vi "PTP.vi"(2 "Run uninterrupted?":bool, 3 "Device Category IN:":string(combo)="Mini" caption="Device Category:", 5 "Sensor Serial No. IN:":string caption="Sensor Serial No.:", 6 "DB Serial No. IN:":string caption="DB Serial No.:") -> (0 "Done!":bool)   [LabVIEW 2019]
doc: "Performs IV measurements according to ATLAS ITk Quality Control Specifications."
uses:
  general_VIs/globals/QC_MeasurementSetup.vi
  general_VIs/globals/QC_RunInformation.vi
  InstrControl/InstrumentSetup.vi
  InstrControl/Switching/Switching.lvclass
  InstrControl/SupplyControl/SupplyControl.lvclass
  InstrControl/ArduinoControl/ArduinoControl.lvclass
  InstrControl/InstrControl.lvclass
  <vilib>/Analysis/NI_AALBase.lvlib
panel:
  out "Measurement Configuration Tab":enum32{"PTP Setup", "PTP Scan"}(tab)
  in  "Test step [V] IN":dbl=10.0 caption="Test Step [V]" format="%.1f"
  in  "Set current limits?":bool
  in  "Current Limit Bias [µA]":dbl=1000.0 min=0.0001 format="%.3f"
  in  "Measurement Configurations":bool
  in  "Bias Voltage [V] IN":dbl=-700.0 caption="Bias Voltage [V]"
  in  "Bias step [V] IN":dbl=10.0 caption="Bias Step [V]" format="%.1f"
  in  "step interval [s] IN":i32=10 caption="Step Interval [s]"
  in  "Continue":bool
  in  "Quit":bool
  in  "Test Final Voltage [V] IN":dbl=-700.0 caption="Test Final Voltage [V]"
  in  "Current Limit SMU [µA]":dbl=1000.0 min=0.0001 format="%.3f"
  out "RH":dbl[](array[numeric]) caption="RH [%]" format="%#.2f"
  out "Temp.":dbl[](array[numeric]) caption="Temp. [°C]" format="%#.2f"
  out "R_eff":dbl[](array[numeric]) caption="Current [nA]"
  out "Volts":dbl[](array[numeric]) caption="Volts [V]"
  out "step interval [s]":i32=10
  out "step [V]":dbl=10.0 format="%.1f"
  out "Final volts [V]":dbl=-700.0 format="%.1f"
  out "Initial volts [V]":dbl format="%.1f"
  out "Igraph":cluster{dbl[], dbl[]}(graph)
  in  "Scales":T1(ring)
  in  "Iscale":enum16{"Ohms", "kiloOhms", "MegaOhms"}(ring)
  out "positive ramp?":bool
  out "DUT Description/Hardware Tab":enum32{"PTP Setup", "PTP Scan"}(tab)
  in  "Structure  Name IN:":string caption="Stucture Name:"
  in  "Test SMU":string(combo)="Keithley 2657A"
  in  "Switching":string(combo)="LXIPXI Switching"
  in  "Hardware Configurations":bool
  in  "User:":string(combo)="Xavi"
  in  "Bias Supply":string(combo)="Keithley 2410"
  in  "Temperature":enum16{"Read Arduino", "Enter manually"}(ring)
  in  "Manufacturer:":string(combo)="Hamamatsu"
  out "Structure Name:":string
  in  "abort":bool
  out "Device Category:":string
  out "DB Serial No.:":string
  out "Current Volts:":dbl format="%.2f"
  in  "quit (no save)":bool
  in  "Quit & Save":bool
  out "Bias On/Off:":bool
  out "STATUS 1":string
  out "Initiated:":string
  out "Sensor No.:":string
  out "No of steps":u32
  out "Current reading No.":u32
  out "Last reading at:":string
  # "Vertical Scale:"
  # "Strip Sensor Testing: PTP"
  # "Measurement Configuration"
  # "PTP Scan parameters:"
  # "Last 5 readings:"
  # "n-4"
  # "n-3"
  # "n-2"
  # "n-1"
  # "n"
  # "DUT Description"
  # "Hardware"
  # "DUT & Test Description:"
  # "Current status:"
  # "Rdg No:"
  # "out of"
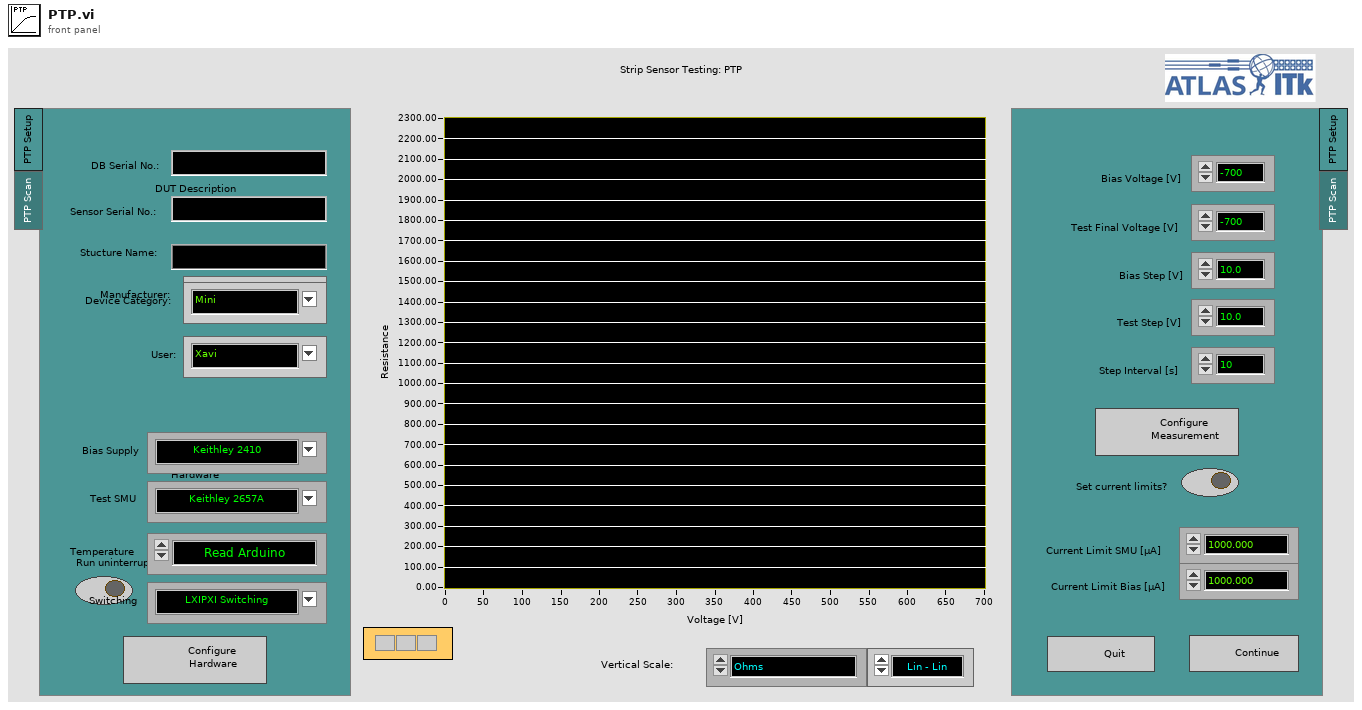
[diagram p1: front panel]
types:
  T1 = enum16{"Lin - Lin", "Log - Lin", "Lin - Log", "Log - log"}
  T2 = enum16{"Supply", "LCR", "Multimeter", "Switching"}
  T3 = enum16{"Reset", "Read Array", "Read Element", "Write Element", "Write Array", "Add Element", "Add Array"}
  T4 = enum16{"Reset", "Ground", "Striptest Bias", "Striptest SMU", "Striptest LCR", "IV", "CV", "Interstrip Cap", "Interstrip Res"}
  T5 = enum16{"Reset", "Ground", "Striptest Bias", "Striptest SMU", "Striptest LCR", "IV", "CV", "Interstrip Cap", "Interstrip Res", "PTP", "Implant Resistance", "Metal Resistance", "Coupling Capacitance"}
  T6 = cluster{"Supply":refnum<class "SupplyControl.lvclass">, "Final Test Voltage [V]":dbl, "Bias Voltage [V]":dbl, "Bias Step Size [V]":dbl, "Step Interval [s]":i32, "Bias Number of Steps":u32, "Ramp down steps [V]":dbl, "Ramp down Interval [s]":i32, "Set Current Limit?":bool, "Current Limit Bias [µA]":dbl, "Temperature Readout":enum16{"Read Arduino", "Enter manually"}, "Arduino":refnum<class "ArduinoControl.lvclass">, "Supply Name":string, "V_breakdown Limit [V]":dbl, "Switching":refnum<class "Switching.lvclass">, "Matrix used?":bool, "Matrix X Channels":cluster{"Bias Supply / SMU LO":i32, "Bias Supply / SMU HI":i32, "CV Box LO":i32, "CV Box HI":i32, "CV Box LO IN":i32, "CV Box HI IN":i32, "Volt meter LO":i32, "Volt meter HI":i32, "Mux1 C1":i32, "Mux1 C2":i32, "Mux2 C1":i32, "Mux2 C2":i32}, "SMU Name":string, "Test Step Size [V] ":dbl, "Test Number of Steps ":u32, "SMU":refnum<class "SupplyControl.lvclass">, "Current Limit SMU [µA] ":dbl, "Structure Name":string}
  T7 = cluster{"Sensor Serial No.:":string, "Wafer Serial No.:":string, "Batch:":string, "Manufacturer:":string, "Device Category:":string, "Database Serial No.:":string, "Date Initiated:":string, "Time Initiated:":string, "Test":string, "Instruments used:":string, "Probeplan used:":string, "End of Run comment:":string, "User:":string}
  T8 = cluster{"Institute":string, "Manufacturers":string[], "Devices":string[], "Serialnumbers Lookup DB":string, "Data directory":string, "Backup & screenshot directory":string, "List of known users":string[], "Measurement switch not used":bool, "Measurement Switch":string, "DUT Switch":string}
  T9 = cluster{"Current Limit":sgl, "KE2410":refnum<class "KE2410.lvclass">}
  T10 = cluster{"Current Limit":sgl, "KE2657A":refnum<class "KE2657A.lvclass">}
  T11 = cluster{"VISA address":refnum<visa-resource-name>, "T sensor":enum16{"SHT", "DS"}, "Arduino":refnum<class "ArduinoControl.lvclass">}
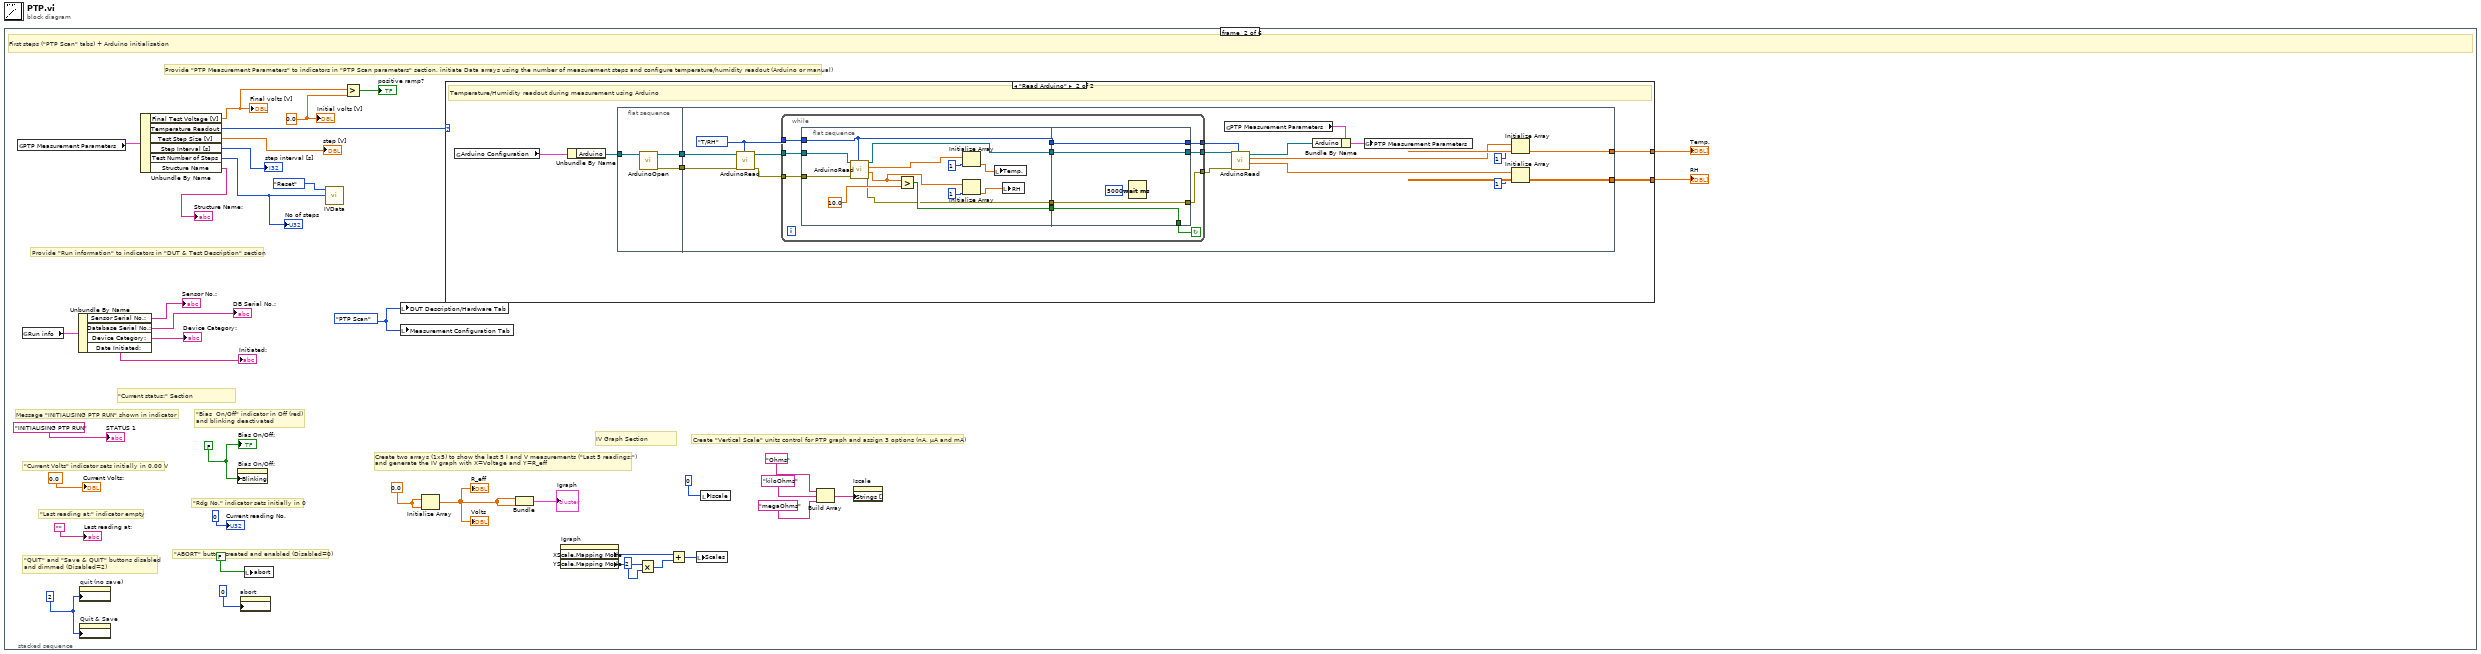
[diagram p0: block diagram]
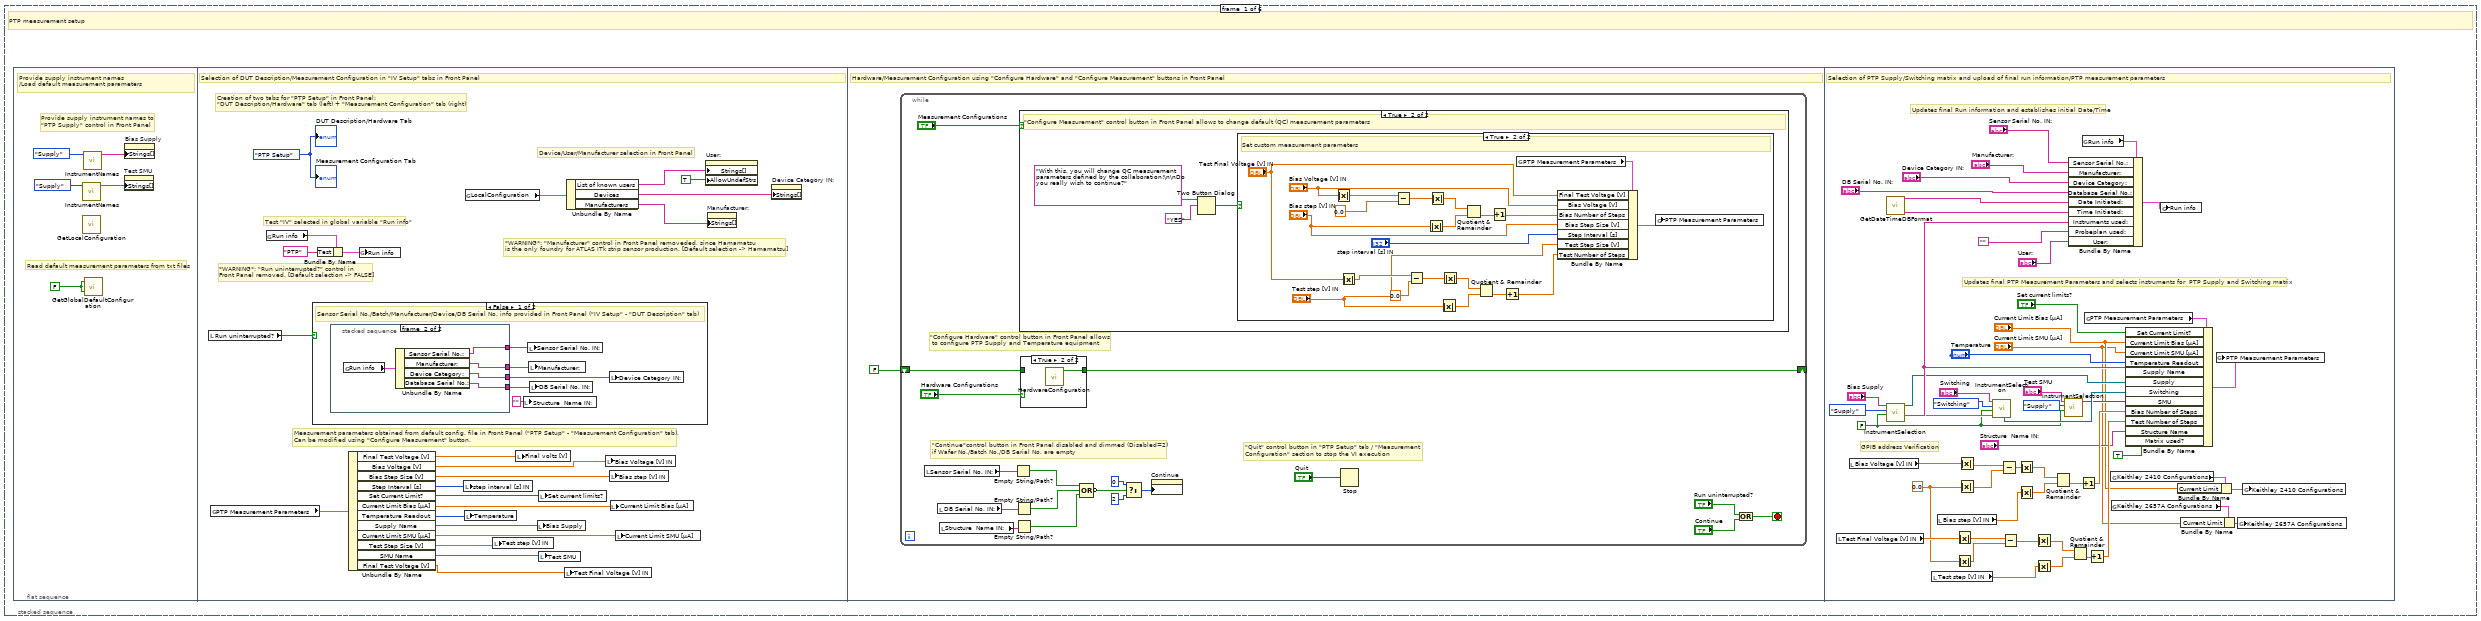
[diagram p2: hidden frame]
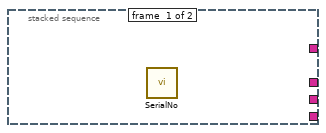
[diagram p3: hidden frame]
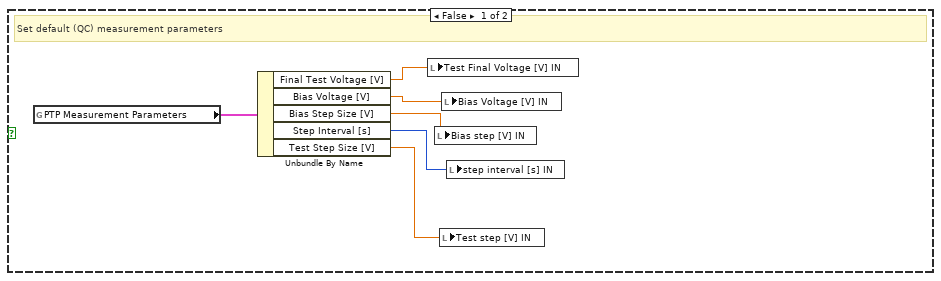
[diagram p6: hidden frame]
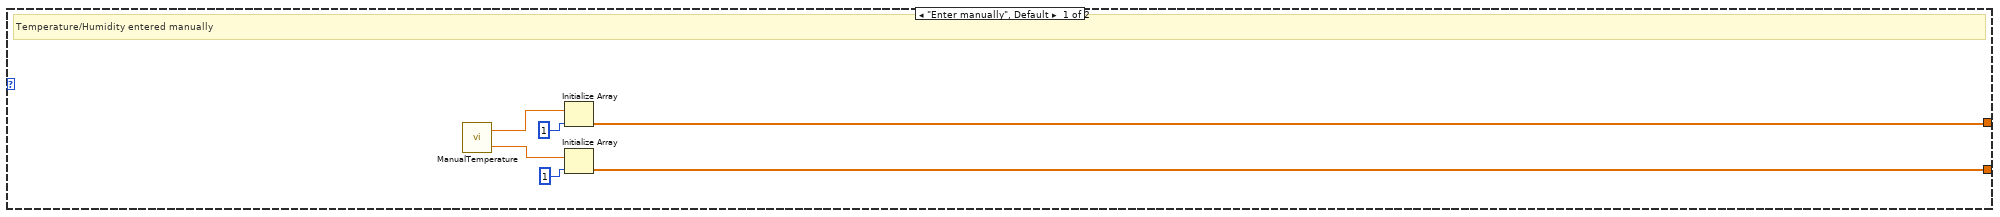
[diagram p8: hidden frame]
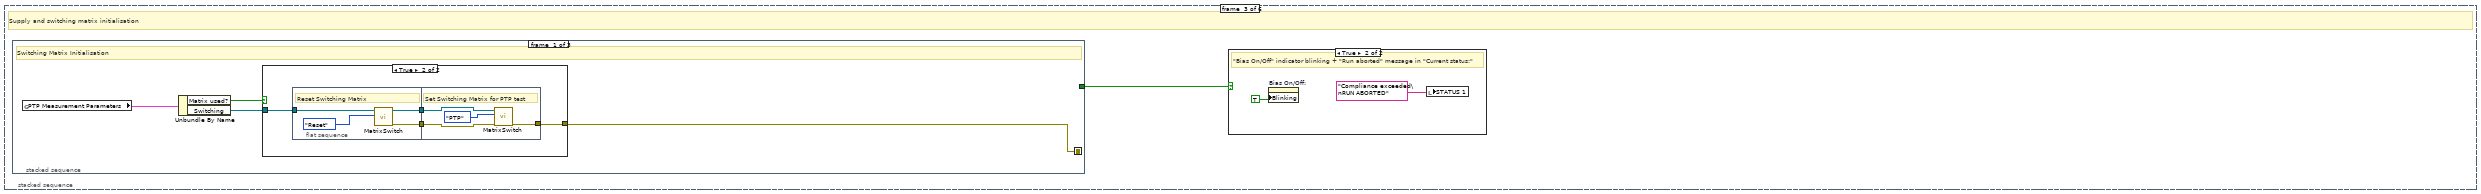
[diagram p9: hidden frame]
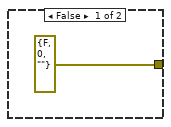
[diagram p10: hidden frame]
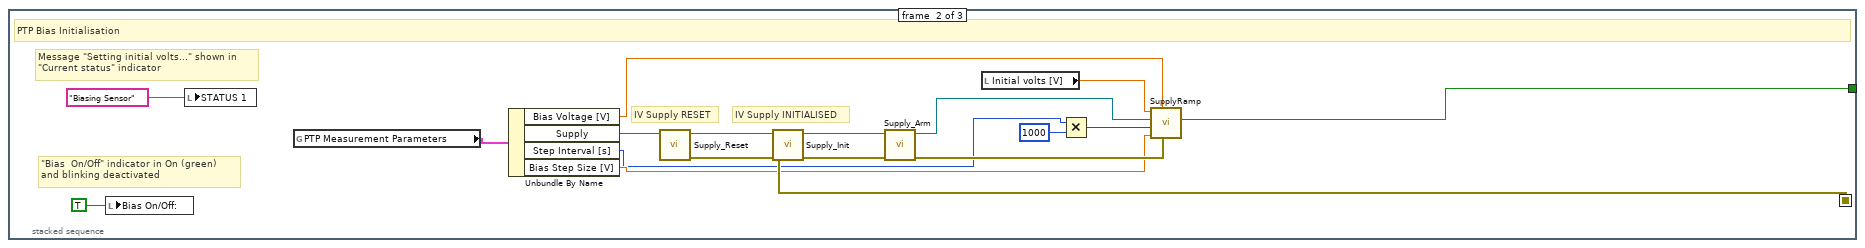
[diagram p11: hidden frame]
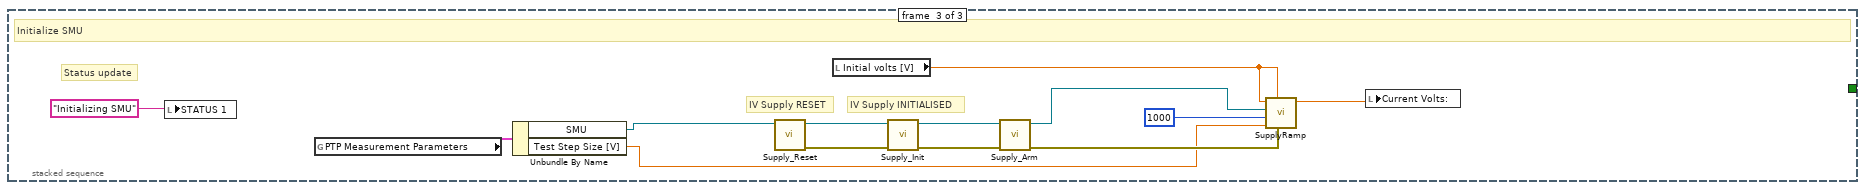
[diagram p12: hidden frame]
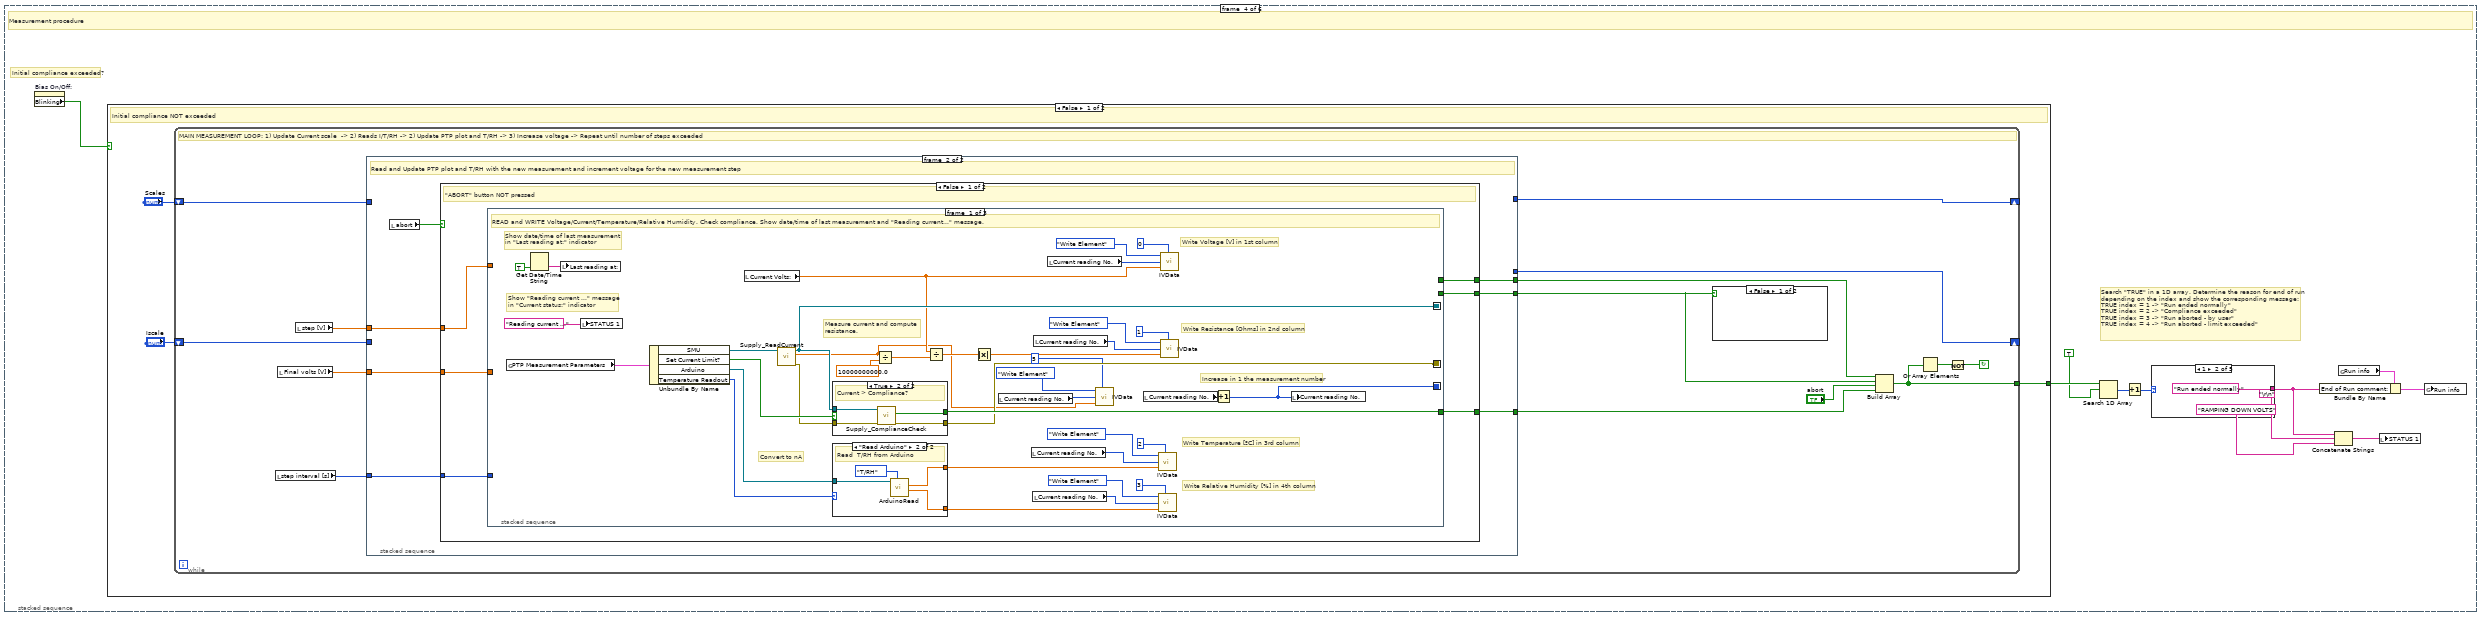
[diagram p14: hidden frame]
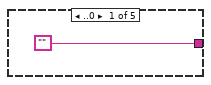
[diagram p15: hidden frame]
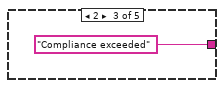
[diagram p16: hidden frame]
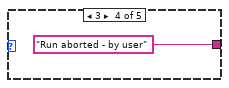
[diagram p17: hidden frame]
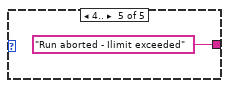
[diagram p18: hidden frame]
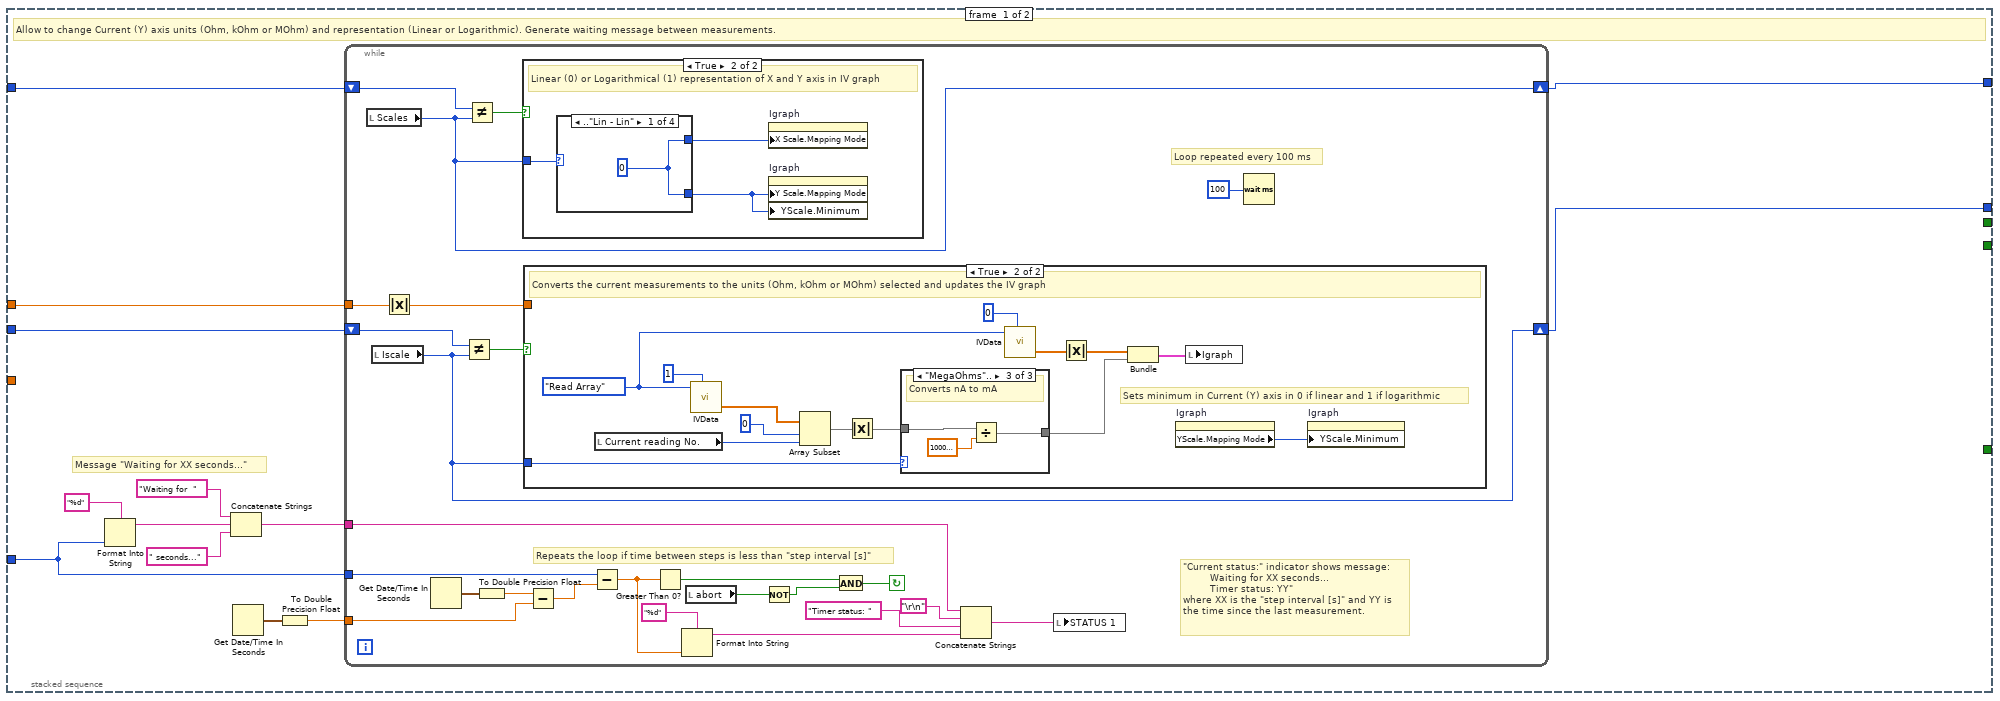
[diagram p19: hidden frame]
diagram:
  n1 = stacked-sequence {
    frame #0 {
      # "PTP measurement setup"
      n2 = flat-sequence {
        frame #0 {
          w5 = FALSE
          # "Read default measurement parameters from txt files"
          # "Provide supply instrument names to \n\"PTP Supply\" control in Front Panel"
          # "Provide supply instrument names\n/Load default measurement parameters"
          n3 = call "InstrumentNames.vi"("Instrument type"=T2."Supply") -> ("Instrument names"=w1:string[])  [unwired: 9 in, 1 out]
          n4 = call "GetLocalConfiguration.vi"() -> ()  [unwired: 3 in, 1 out]
          n5 = call "InstrumentNames.vi"("Instrument type"=T2."Supply") -> ("Instrument names"=w3:string[])  [unwired: 9 in, 1 out]
          n6 = call "GetGlobalDefaultConfiguration.vi"("DO NOT override instruments"=w5, "Read defaults?"=w5) -> ()  [unwired: 1 in, 1 out]
          n7 = property on="Test SMU" class="CmbBox"("Strings[]"=w1) -> ()  [unwired: 2 in, 2 out]
          n8 = property on="Bias Supply" class="CmbBox"("Strings[]"=w3) -> ()  [unwired: 2 in, 2 out]
        }
        frame #1 {
          w16 = enum32{"PTP Setup", "PTP Scan"}."PTP Setup" ("Tab Control")
          # "Device/User/Manufacturer selection in Front Panel"
          # "*WARNING*: \"Manufacturer\" control in Front Panel removeded, since Hamamatsu \nis the only foundry for ATLAS ITk strip sensor production. [Default selection -> Hamamatsu]"
          # "Measurement parameters obtained from default config. file in Front Panel (\"PTP Setup\" - \"Measurement Configuration\" tab).\nCan be modified using \"Configure Measurement\" button."
          # "Test \"IV\" selected in global variable \"Run info\""
          # "Creation of two tabs for \"PTP Setup\" in Front Panel:\n\"DUT Description/Hardware\" tab (left) + \"Measurement Configuration\" tab (right)"
          # "*WARNING*: \"Run uninterrupted?\" control in \nFront Panel removed. [Default selection -> FALSE]"
          # "Selection of DUT Description/Measurement Configuration in \"IV Setup\" tabs in Front Panel"
          n9 = local read "Run uninterrupted?"() -> (w20:bool)
          n10 = global read "QC_MeasurementSetup.vi" "PTP Measurement Parameters"() -> (w26:T6)
          n11 = global read "QC_RunInformation.vi" "Run info"() -> (w19:T7)
          n12 = case shown="False" w20 {
            frame False {
              # "Sensor Serial No./Batch/Manufacturer/Device/DB Serial No. info provided in Front Panel (\"IV Setup\" - \"DUT Description\" tab)"
              n13 = stacked-sequence {
                tunnel: [_ w38] -> w32
                tunnel: [_ w37] -> w31
                tunnel: [_ w36] -> w33
                tunnel: [_ w34] -> w30
                frame #0 {
                  n14 = call "SerialNo.vi"() -> ()  [unwired: 5 in, 1 out]
                }
                frame #1 {
                  n15 = global read "QC_RunInformation.vi" "Run info"() -> (w35:T7)
                  n16 = Unbundle By Name(w35) -> ("Sensor Serial No.:"=w38:string, "Manufacturer:"=w37:string, "Device Category:"=w36:string, "Database Serial No.:"=w34:string)
                }
              }
              n17 = local write "Structure  Name IN:"("" ("Structure Name")) -> ()
              n18 = local write "Sensor Serial No. IN:"(w32) -> ()
              n19 = local write "Manufacturer:"(w31) -> ()
              n20 = local write "DB Serial No. IN:"(w30) -> ()
              n21 = local write "Device Category IN:"(w33) -> ()
            }
            frame True {
            }
          }
          n22 = Bundle By Name(cluster=w19, "Test"="PTP") -> (w17:T7)
          n23 = Unbundle By Name(w26) -> ("Final Test Voltage [V]"=w11:dbl, "Bias Voltage [V]"=w10:dbl, "Bias Step Size [V]"=w14:dbl, "Step Interval [s]"=w15:i32, "Set Current Limit?"=w25:bool, "Current Limit Bias [µA]"=w24:dbl, "Temperature Readout"=w28:enum16{"Read Arduino", "Enter manually"}, "Supply Name"=w27:string, "Current Limit SMU [µA]"=w6:dbl, "Test Step Size [V]"=w9:dbl, "SMU Name"=w8:string, "Final Test Voltage [V]"=w7:dbl)
          n24 = global write "QC_RunInformation.vi" "Run info"(w17) -> ()
          n25 = local write "step interval [s] IN"(w15) -> ()
          n26 = local write "Temperature"(w28) -> ()
          n27 = global read "QC_RunInformation.vi" "LocalConfiguration"() -> (w23:T8)
          n28 = local write "Test step [V] IN"(w9) -> ()
          n29 = local write "Final volts [V]"(w11) -> ()
          n30 = local write "Bias Supply"(w27) -> ()
          n31 = local write "Set current limits?"(w25) -> ()
          n32 = local write "Test SMU"(w8) -> ()
          n33 = local write "Test Final Voltage [V] IN"(w7) -> ()
          n34 = Unbundle By Name(w23) -> ("List of known users"=w22:string[], "Devices"=w13:string[], "Manufacturers"=w12:string[])
          n35 = local write "Bias Voltage [V] IN"(w10) -> ()
          n36 = local write "Bias step [V] IN"(w14) -> ()
          n37 = local write "Current Limit Bias [µA]"(w24) -> ()
          n38 = local write "Current Limit SMU [µA]"(w6) -> ()
          n39 = property on="User:" class="CmbBox"("Strings[]"=w22, "AllowUndefStrs"=TRUE) -> ()  [unwired: 2 in, 2 out]
          n40 = property on="Manufacturer:" class="CmbBox"("Strings[]"=w12) -> ()  [unwired: 2 in, 2 out]
          n41 = property on="Device Category IN:" class="CmbBox"("Strings[]"=w13) -> ()  [unwired: 2 in, 2 out]
          "DUT Description/Hardware Tab" <- w16
          "Measurement Configuration Tab" <- w16
        }
        frame #2 {
          # "Hardware/Measurement Configuration using \"Configure Hardware\" and \"Configure Measurement\" buttons in Front Panel"
          n42 = while {
            shift-right: [w49] -> _
            shift-left: FALSE -> [w48]
            stop <- w45 stop-if-true
            # "\"Continue\"control button in Front Panel disabled and dimmed (Disabled=2) \nif Wafer No./Batch No./DB Serial No. are empty"
            # "\"Configure Hardware\" control button in Front Panel allows\n to configure PTP Supply and Temperature equipment"
            # "\"Quit\" control button in \"PTP Setup\" tab / \"Measurement \nConfiguration\" section to stop the VI execution"
            n43 = local read "Sensor Serial No. IN:"() -> (w56:string)
            n44 = local read "DB Serial No. IN:"() -> (w43:string)
            n45 = local read "Structure  Name IN:"() -> (w41:string)
            n46 = Empty String/Path?(string/path=w56) -> (empty?=w55:bool)
            n47 = Empty String/Path?(string/path=w43) -> (empty?=w42:bool)
            n48 = Empty String/Path?(string/path=w41) -> (empty?=w40:bool)
            n49 = case shown="True" "Measurement Configurations" {
              frame False {
              }
              frame True {
                # "\"Configure Measurement\" control button in Front Panel allows to change default (QC) measurement parameters"
                n50 = Two Button Dialog(message="With this, you will change QC measurement parameters defined by the collaboration!\n\nDo you really wish to continue?", 2:"YES") -> (T button?=w58:bool)  [unwired: 1 in]
                n51 = case shown="True" w58 {
                  frame False {
                    # "Set default (QC) measurement parameters"
                    n52 = global read "QC_MeasurementSetup.vi" "PTP Measurement Parameters"() -> (w66:T6)
                    n53 = Unbundle By Name(w66) -> ("Final Test Voltage [V]"=w64:dbl, "Bias Voltage [V]"=w65:dbl, "Bias Step Size [V]"=w63:dbl, "Step Interval [s]"=w62:i32, "Test Step Size [V]"=w61:dbl)
                    n54 = local write "Test Final Voltage [V] IN"(w64) -> ()
                    n55 = local write "Bias step [V] IN"(w63) -> ()
                    n56 = local write "Test step [V] IN"(w61) -> ()
                    n57 = local write "Bias Voltage [V] IN"(w65) -> ()
                    n58 = local write "step interval [s] IN"(w62) -> ()
                  }
                  frame True {
                    # "Set custom measurement parameters"
                    n59 = Absolute Value(x="Bias Voltage [V] IN") -> (abs(x)=w85:dbl)
                    n60 = Absolute Value(x="Test Final Voltage [V] IN") -> (abs(x)=w72:dbl)
                    n61 = Subtract(x=w85, y=0.0) -> (x-y=w81:dbl)
                    n62 = Subtract(x=w72, y=0.0) -> (x-y=w75:dbl)
                    n63 = Absolute Value(x="Bias step [V] IN") -> (abs(x)=w82:dbl)
                    n64 = Absolute Value(x=w81) -> (abs(x)=w83:dbl)
                    n65 = Absolute Value(x="Test step [V] IN") -> (abs(x)=w76:dbl)
                    n66 = Absolute Value(x=w75) -> (abs(x)=w77:dbl)
                    n67 = Quotient & Remainder(x=w83, y=w82) -> (floor(x/y)=w80:dbl)  [unwired: 1 out]
                    n68 = Quotient & Remainder(x=w77, y=w76) -> (floor(x/y)=w74:dbl)  [unwired: 1 out]
                    n69 = Increment(x=w80) -> (x+1=w79:dbl)
                    n70 = Increment(x=w74) -> (x+1=w67:dbl)
                    n71 = global read "QC_MeasurementSetup.vi" "PTP Measurement Parameters"() -> (w87:T6)
                    n72 = Bundle By Name(cluster=w87, "Final Test Voltage [V]"="Test Final Voltage [V] IN", "Bias Voltage [V]"="Bias Voltage [V] IN", "Bias Number of Steps"=w79, "Bias Step Size [V]"="Bias step [V] IN", "Step Interval [s]"="step interval [s] IN", "Test Step Size [V]"="Test step [V] IN", "Test Number of Steps"=w67) -> (w86:T6)
                    n73 = global write "QC_MeasurementSetup.vi" "PTP Measurement Parameters"(w86) -> ()
                  }
                }
              }
            }
            n74 = case shown="True" "Hardware Configurations" {
              tunnel: [w88 w89] -> w49
              tunnel: w48 -> [w88 _]
              frame False {
              }
              frame True {
                n75 = call "HardwareConfiguration.vi"() -> ("configured?"=w89:bool)  [unwired: 11 in]
              }
            }
            n76 = Compound Arithmetic op=OR(w55, w42, w40) -> (invert w54:bool)
            n77 = Select(t=0, s=w54, f=2) -> (s? t:f=w51:i32)
            n78 = property on="Continue" class="Bool"("DisabledEnum"=w51) -> ()  [unwired: 2 in, 2 out]
            n79 = Stop(stop? (T)="Quit") -> ()
            n80 = Or(x="Run uninterrupted?", y="Continue") -> (x .or. y?=w45:bool)
          }
        }
        frame #3 {
          w104 = 0.0 ("x")
          w100 = FALSE
          # "GPIB address Verification"
          # "Updates final PTP Measurement Parameters and selects instruments for  PTP Supply and Switching matrix"
          # "Updates final Run information and establishes initial Date/Time"
          # "Selection of PTP Supply/Switching matrix and upload of final run information/PTP measurement parameters"
          n81 = local read "Test Final Voltage [V] IN"() -> (w105:dbl)
          n82 = local read "Bias Voltage [V] IN"() -> (w115:dbl)
          n83 = call "InstrumentSelection.vi"("Verify GPIB address"=w100, "Instrument type"=T2."Supply", "Instrument name IN"="Bias Supply") -> ("error out"=w128:errorcluster, "Instrument name OUT"=w131:string, "Supply"=w130:refnum<class "SupplyControl.lvclass">)  [unwired: 3 in, 3 out]
          n84 = call "GetDateTimeDBFormat.vi"() -> ("Time in 24h format, e.g. 13:40:54"=w90:string, "Abbreviated Date, e.g. 13 Nov 2020"=w91:string)  [unwired: 10 in]
          n85 = local read "Test step [V] IN"() -> (w103:dbl)
          n86 = local read "Bias step [V] IN"() -> (w116:dbl)
          n87 = Absolute Value(x=w105) -> (abs(x)=w111:dbl)
          n88 = Absolute Value(x=w104) -> (abs(x)=w110:dbl)
          n89 = Absolute Value(x=w115) -> (abs(x)=w122:dbl)
          n90 = Absolute Value(x=w104) -> (abs(x)=w121:dbl)
          n91 = call "InstrumentSelection.vi"("error in (no error)"=w128, "Verify GPIB address"=w100, "Instrument type"=T2."Switching", "Instrument name IN"="Switching") -> ("Switching"=w127:refnum<class "Switching.lvclass">)  [unwired: 2 in, 5 out]
          n92 = Subtract(x=w122, y=w121) -> (x-y=w118:dbl)
          n93 = Subtract(x=w111, y=w110) -> (x-y=w107:dbl)
          n94 = Absolute Value(x=w118) -> (abs(x)=w120:dbl)
          n95 = Absolute Value(x=w116) -> (abs(x)=w119:dbl)
          n96 = Absolute Value(x=w107) -> (abs(x)=w109:dbl)
          n97 = Absolute Value(x=w103) -> (abs(x)=w108:dbl)
          n98 = Quotient & Remainder(x=w120, y=w119) -> (floor(x/y)=w117:dbl)  [unwired: 1 out]
          n99 = call "InstrumentSelection.vi"("Verify GPIB address"=w100, "Instrument type"=T2."Supply", "Instrument name IN"="Test SMU") -> ("Supply"=w112:refnum<class "SupplyControl.lvclass">)  [unwired: 3 in, 5 out]
          n100 = Quotient & Remainder(x=w109, y=w108) -> (floor(x/y)=w106:dbl)  [unwired: 1 out]
          n101 = Increment(x=w117) -> (x+1=w102:dbl)
          n102 = global read "QC_RunInformation.vi" "Run info"() -> (w139:T7)
          n103 = Bundle By Name(cluster=w139, "Sensor Serial No.:"="Sensor Serial No. IN:", "Manufacturer:"="Manufacturer:", "Device Category:"="Device Category IN:", "Database Serial No.:"="DB Serial No. IN:", "Date Initiated:"=w91, "Time Initiated:"=w90, "Instruments used:"=w131, "Probeplan used:"="", "User:"="User:") -> (w138:T7)
          n104 = global read "QC_MeasurementSetup.vi" "PTP Measurement Parameters"() -> (w141:T6)
          n105 = Increment(x=w106) -> (x+1=w101:dbl)
          n106 = global read "InstrumentSetup.vi" "Keithley 2410 Configurations"() -> (w98:T9)
          n107 = global read "InstrumentSetup.vi" "Keithley 2657A Configurations"() -> (w95:T10)
          n108 = Bundle By Name(cluster=w141, "Set Current Limit?"="Set current limits?", "Current Limit Bias [µA]"="Current Limit Bias [µA]", "Current Limit SMU [µA]"="Current Limit SMU [µA]", "Temperature Readout"="Temperature", "Supply Name"=w131, "Supply"=w130, "Switching"=w127, "SMU"=w112, "Bias Number of Steps"=w102, "Test Number of Steps"=w101, "Structure Name"="Structure  Name IN:", "Matrix used?"=TRUE) -> (w142:T6)
          n109 = global write "QC_RunInformation.vi" "Run info"(w138) -> ()
          n110 = Bundle By Name(cluster=w98, "Current Limit"="Current Limit Bias [µA]") -> (w97:T9)
          n111 = Bundle By Name(cluster=w95, "Current Limit"="Current Limit SMU [µA]") -> (w94:T10)
          n112 = global write "QC_MeasurementSetup.vi" "PTP Measurement Parameters"(w142) -> ()
          n113 = global write "InstrumentSetup.vi" "Keithley 2657A Configurations"(w94) -> ()
          n114 = global write "InstrumentSetup.vi" "Keithley 2410 Configurations"(w97) -> ()
        }
      }
    }
    frame #1 {
      w144 = 0.0 ("y")
      w150 = enum32{"PTP Setup", "PTP Scan"}."PTP Scan" ("Tab Control")
      w165 = 2
      w171 = 0.0
      w164 = FALSE ("Visible")
      # "IV Graph Section"
      # "\"Current status:\" Section"
      # "Create two arrays (1x5) to show the last 5 I and V measurements (\"Last 5 readings:\") \nand generate the IV graph with X=Voltage and Y=R_eff"
      # "\"Bias  On/Off\" indicator in Off (red)\nand blinking deactivated"
      # "\"Rdg No.\" indicator sets initially in 0"
      # "\"ABORT\" button created and enabled (Disabled=0)"
      # "\"Current Volts\" indicator sets initially in 0.00 V"
      # "\"Last reading at:\" indicator empty"
      # "\"QUIT\" and \"Save & QUIT\" buttons disabled\nand dimmed (Disabled=2)"
      # "Message \"INITIALISING PTP RUN\" shown in indicator"
      # "Create \"Vertical Scale\" units control for PTP graph and assign 3 options (nA, µA and mA)"
      # "Provide \"Run information\" to indicators in \"DUT & Test Description\" section"
      # "Provide \"PTP Measurement Parameters\" to indicators in \"PTP Scan parameters\" section, initiate Data arrays using the number of measurement steps and configure temperature/humidity readout (Arduino or manual)"
      # "First steps (\"PTP Scan\" tabs) + Arduino initialisation"
      n115 = global read "QC_MeasurementSetup.vi" "PTP Measurement Parameters"() -> (w155:T6)
      n116 = global read "QC_RunInformation.vi" "Run info"() -> (w180:T7)
      n117 = Unbundle By Name(w180) -> ("Sensor Serial No.:"=→"Sensor No.:":string, "Database Serial No.:"=→"DB Serial No.:":string, "Device Category:"=→"Device Category:":string, "Date Initiated:"=→"Initiated:":string)
      n118 = property on="quit (no save)" class="Bool"("DisabledEnum"=w165) -> ()  [unwired: 2 in, 2 out]
      n119 = property on="Quit & Save" class="Bool"("DisabledEnum"=w165) -> ()  [unwired: 2 in, 2 out]
      n120 = Unbundle By Name(w155) -> ("Final Test Voltage [V]"=w145:dbl, "Temperature Readout"=w148:enum16{"Read Arduino", "Enter manually"}, "Test Step Size [V]"=→"step [V]":dbl, "Step Interval [s]"=→"step interval [s]":i32, "Test Number of Steps"=w146:u32, "Structure Name"=→"Structure Name:":string)
      "No of steps" <- w146
      "Final volts [V]" <- w145
      n121 = property on="Bias On/Off:" class="Bool (strict)"("Blinking"=w164) -> ()  [unwired: 2 in, 2 out]
      n122 = property on="abort" class="Bool (strict)"("DisabledEnum"=0) -> ()  [unwired: 2 in, 2 out]
      n123 = local write "abort"(FALSE) -> ()
      n124 = call "IVData.vi"("Action"=T3."Reset", "Array Size / Index"=w146) -> ()  [unwired: 3 in, 2 out]
      n125 = Greater?(x=w145, y=w144) -> (0:→"positive ramp?":bool)
      n126 = local write "DUT Description/Hardware Tab"(w150) -> ()
      n127 = local write "Measurement Configuration Tab"(w150) -> ()
      n128 = Initialize Array(w171, w171) -> (w151:dbl[])
      "Volts" <- w151
      "R_eff" <- w151
      n129 = case shown="\"Read Arduino\"" w148 {
        tunnel: [w186 w193] -> w168
        tunnel: [w183 w192] -> w156
        frame "Enter manually", Default {
          # "Temperature/Humidity entered manually"
          n130 = call "ManualTemperature.vi"() -> ("Humidity [%] out"=w182:dbl, "Temperature [°C] out"=w187:dbl)
          n131 = Initialize Array(w187, 1) -> (w186:dbl[])
          n132 = Initialize Array(w182, 1) -> (w183:dbl[])
        }
        frame "Read Arduino" {
          # "Temperature/Humidity readout during measurement using Arduino"
          n133 = global read "InstrumentSetup.vi" "Arduino Configuration"() -> (w189:T11)
          n134 = Unbundle By Name(w189) -> ("Arduino"=w188:refnum<class "ArduinoControl.lvclass">)
          n135 = flat-sequence {
            tunnel: [w194] -> w191
            tunnel: [w196] -> w190
            tunnel: w188 -> [w195]
            tunnel: [w213] -> w193
            tunnel: [w210] -> w192
            tunnel: w191 -> [w204]
            tunnel: w190 -> [w203]
            frame #0 {
              n136 = call "ArduinoOpen.vi"("ArduinoControl in"=w195) -> ("error out"=w196:errorcluster, "ArduinoControl out"=w194:refnum<class "ArduinoControl.lvclass">)  [unwired: 9 in]
            }
            frame #1 {
              w200 = enum16{"T/RH", "Interlock", "Edgesense"}."T/RH" ("Arduino function")
              n137 = call "ArduinoRead.vi"("Arduino function"=w200, "error in (no error)"=w203, "ArduinoControl in"=w204) -> ("error out"=w201:errorcluster, "ArduinoControl out"=w202:refnum<class "ArduinoControl.lvclass">)  [unwired: 3 in, 4 out]
              n138 = while {
                tunnel: w202 -> [w215]
                tunnel: w201 -> [w214]
                tunnel: w200 -> [w224]
                tunnel: [w222] -> w197
                tunnel: [w218] -> w199
                tunnel: [w216] -> w198
                stop <- w221 continue-if-true
                n139 = flat-sequence {
                  tunnel: w215 -> [w236]
                  tunnel: w214 -> [w235]
                  tunnel: w224 -> [w234]
                  tunnel: [w234] -> w223
                  tunnel: [w233] -> w220
                  tunnel: [w232] -> w219
                  tunnel: [w231] -> w217
                  tunnel: [w242] -> w222
                  tunnel: w223 -> [w242]
                  tunnel: [w241] -> w221
                  tunnel: w220 -> [w241]
                  tunnel: [w239] -> w218
                  tunnel: w219 -> [w239]
                  tunnel: [w238] -> w216
                  tunnel: w217 -> [w238]
                  frame #0 {
                    n140 = call "ArduinoRead.vi"("Arduino function"=w234, "error in (no error)"=w235, "ArduinoControl in"=w236) -> ("error out"=w232:errorcluster, "rel. Humidity [%]"=w227:dbl, "Temperature [°C]"=w228:dbl, "ArduinoControl out"=w231:refnum<class "ArduinoControl.lvclass">)  [unwired: 3 in, 2 out]
                    n141 = Greater?(x=w227, y=10.0 ("Start Humidity")) -> (0:w233:bool)
                    n142 = Initialize Array(w228, 1) -> (w225:dbl[])
                    n143 = Initialize Array(w227, 1) -> (w226:dbl[])
                    n144 = local write "Temp."(w225) -> ()
                    n145 = local write "RH"(w226) -> ()
                  }
                  frame #1 {
                    n146 = Wait (ms)(milliseconds to wait=u32 5000) -> ()  [unwired: 1 out]
                  }
                }
              }
              n147 = global read "QC_MeasurementSetup.vi" "PTP Measurement Parameters"() -> (w206:T6)
              n148 = call "ArduinoRead.vi"("Arduino function"=w197, "error in (no error)"=w199, "ArduinoControl in"=w198) -> ("rel. Humidity [%]"=w208:dbl, "Temperature [°C]"=w209:dbl, "ArduinoControl out"=w207:refnum<class "ArduinoControl.lvclass">)  [unwired: 3 in, 3 out]
              n149 = Bundle By Name(cluster=w206, "Arduino"=w207) -> (w205:T6)
              n150 = global write "QC_MeasurementSetup.vi" "PTP Measurement Parameters"(w205) -> ()
              n151 = Initialize Array(w209, 1) -> (w213:dbl[])
              n152 = Initialize Array(w208, 1) -> (w210:dbl[])
            }
          }
        }
      }
      "Temp." <- w168
      "RH" <- w156
      n153 = Bundle(w151, w151) -> (→"Igraph":cluster{dbl[], dbl[]})  [unwired: 1 in]
      n154 = property on="Igraph" class="XYGraph (strict)"() -> ("XScale.Mapping Mode"=w159:u8, "YScale.Mapping Mode"=w158:u8)  [unwired: 2 in, 2 out]
      n155 = Multiply(x=w158, y=2) -> (x*y=w161:i32)
      n156 = Add(x=w159, y=w161) -> (x+y=w157:i32)
      n157 = local write "Scales"(w157) -> ()
      n158 = local write "Iscale"(u16 0 ("Scale")) -> ()
      n159 = Build Array("Ohms", "kiloOhms", "megaOhms") -> (w177:string[])
      n160 = property on="Iscale" class="Enum (strict)"("Strings []"=w177) -> ()  [unwired: 2 in, 2 out]
      "STATUS 1" <- "INITIALISING PTP RUN"
      "Initial volts [V]" <- w144
      "Bias On/Off:" <- w164
      "Last reading at:" <- ""
      "Current reading No." <- u32 0 ("Current reading No.")
      "Current Volts:" <- 0.0 ("Current Volts:")
    }
    frame #2 {
      # "Supply and switching matrix initialisation"
      n161 = stacked-sequence {
        seq-local: [w245 _ _] -> [_ w267 _]
        tunnel: [_ w268 _] -> w243
        frame #0 {
          # "Switching Matrix Initialisation"
          n162 = global read "QC_MeasurementSetup.vi" "PTP Measurement Parameters"() -> (w244:T6)
          n163 = Unbundle By Name(w244) -> ("Matrix used?"=w247:bool, "Switching"=w246:refnum<class "Switching.lvclass">)
          n164 = case shown="True" w247 {
            tunnel: w246 -> [_ w249]
            tunnel: [errorcluster {"status"=FALSE, "code"=0, "source"=""} ("error constant") w250] -> w245
            frame False {
            }
            frame True {
              n165 = flat-sequence {
                tunnel: [w256] -> w252
                tunnel: [w255] -> w251
                tunnel: w249 -> [w254]
                tunnel: w252 -> [w260]
                tunnel: w251 -> [w259]
                tunnel: [w258] -> w250
                frame #0 {
                  # "Reset Switching Matrix"
                  n166 = call-dynamic "MatrixSwitch.vi"("Action"=T4."Reset", "Switching in"=w254) -> ("error out"=w256:errorcluster, "Switching out"=w255:refnum<class "Switching.lvclass">)  [unwired: 7 in, 1 out]
                }
                frame #1 {
                  # "Set Switching Matrix for PTP test"
                  n167 = call-dynamic "MatrixSwitch.vi"("error in (no error)"=w260, "Action"=T5."PTP", "Switching in"=w259) -> ("error out"=w258:errorcluster)  [unwired: 6 in, 2 out]
                }
              }
            }
          }
        }
        frame #1 {
          # "IV Supply INITIALISED"
          # "IV Supply RESET"
          # "Message \"Setting initial volts...\" shown in \n\"Current status\" indicator"
          # "\"Bias  On/Off\" indicator in On (green)\nand blinking deactivated"
          # "PTP Bias Initialisation"
          n168 = local write "Bias On/Off:"(TRUE ("Compliance?")) -> ()
          n169 = local write "STATUS 1"("Biasing Sensor" ("STATUS 1")) -> ()
          n170 = global read "QC_MeasurementSetup.vi" "PTP Measurement Parameters"() -> (w274:T6)
          n171 = Unbundle By Name(w274) -> ("Bias Voltage [V]"=w265:dbl, "Supply"=w271:refnum<class "SupplyControl.lvclass">, "Step Interval [s]"=w263:i32, "Bias Step Size [V]"=w266:dbl)
          n172 = call-dynamic "Supply_Reset.vi"("error in (no error)"=w267, "SupplyControl in"=w271) -> ("error out"=w276:errorcluster, "SupplyControl out"=w278:refnum<class "SupplyControl.lvclass">)  [unwired: 8 in]
          n173 = call-dynamic "Supply_Init.vi"("error in (no error)"=w276, "SupplyControl in"=w278) -> ("error out"=w275:errorcluster, "SupplyControl out"=w277:refnum<class "SupplyControl.lvclass">)  [unwired: 8 in]
          n174 = call-dynamic "Supply_Arm.vi"("error in (no error)"=w275, "SupplyControl in"=w277) -> ("error out"=w269:errorcluster, "SupplyControl out"=w270:refnum<class "SupplyControl.lvclass">)  [unwired: 8 in]
          n175 = local read "Initial volts [V]"() -> (w261:dbl)
          n176 = Multiply(x=w263, y=1000) -> (x*y=w262:i32)
          n177 = call "SupplyRamp.vi"("error in"=w269, "Requested Voltage"=w265, "Step Size"=w266, "Step Delay"=w262, "Supply IN"=w270, "Starting Voltage"=w261) -> ("Compliance exceeded"=w268:bool)  [unwired: 2 in, 3 out]
        }
        frame #2 {
          # "Status update"
          # "IV Supply INITIALISED"
          # "IV Supply RESET"
          # "Initialize SMU"
          n178 = local write "STATUS 1"("Initializing SMU" ("STATUS 1")) -> ()
          n179 = global read "QC_MeasurementSetup.vi" "PTP Measurement Parameters"() -> (w291:T6)
          n180 = Unbundle By Name(w291) -> ("SMU"=w283:refnum<class "SupplyControl.lvclass">, "Test Step Size [V]"=w281:dbl)
          n181 = call-dynamic "Supply_Reset.vi"("SupplyControl in"=w283) -> ("error out"=w288:errorcluster, "SupplyControl out"=w290:refnum<class "SupplyControl.lvclass">)  [unwired: 9 in]
          n182 = local read "Initial volts [V]"() -> (w282:dbl)
          n183 = call-dynamic "Supply_Init.vi"("error in (no error)"=w288, "SupplyControl in"=w290) -> ("error out"=w287:errorcluster, "SupplyControl out"=w289:refnum<class "SupplyControl.lvclass">)  [unwired: 8 in]
          n184 = call-dynamic "Supply_Arm.vi"("error in (no error)"=w287, "SupplyControl in"=w289) -> ("error out"=w285:errorcluster, "SupplyControl out"=w286:refnum<class "SupplyControl.lvclass">)  [unwired: 8 in]
          n185 = call "SupplyRamp.vi"("error in"=w285, "Requested Voltage"=w282, "Step Size"=w281, "Step Delay"=u32 1000, "Supply IN"=w286, "Starting Voltage"=w282) -> ("Current Voltage"=w280:dbl)  [unwired: 2 in, 3 out]
          n186 = local write "Current Volts:"(w280) -> ()
        }
      }
      n187 = case shown="True" w243 {
        frame False {
        }
        frame True {
          # "\"Bias On/Off\" indicator blinking + \"Run aborted\" message in \"Current status:\""
          n188 = property on="Bias On/Off:" class="Bool (strict)"("Blinking"=TRUE) -> ()  [unwired: 2 in, 2 out]
          n189 = local write "STATUS 1"("Compliance exceeded\nRUN ABORTED") -> ()
        }
      }
    }
    frame #3 {
      # "Search \"TRUE\" in a 1D array. Determine the reason for end of run \ndepending on the index and show the corresponding message:\nTRUE index = 1 -> \"Run ended normally\"\nTRUE index = 2 -> \"Compliance exceeded\"\nTRUE index = 3 -> \"Run aborted - by user\"\nTRUE index = 4 -> \"Run aborted - limit exceeded\""
      # "Initial compliance exceeded?"
      # "Measurement procedure"
      n190 = property on="Bias On/Off:" class="Bool (strict)"() -> ("Blinking"=w304:bool)  [unwired: 2 in, 2 out]
      n191 = case shown="False" w304 {
        tunnel: [w312 w557] -> w303
        frame False {
          # "Initial compliance NOT exceeded"
          n192 = while {
            shift-left: "Iscale" -> [w322]
            shift-right: [w321] -> _
            shift-left: "Scales" -> [w323]
            shift-right: [w324] -> _
            tunnel: [w320] -> w312
            stop <- w325 continue-if-true
            # "MAIN MEASUREMENT LOOP: 1) Update Current scale  -> 2) Reads I/T/RH -> 2) Update PTP plot and T/RH -> 3) Increase voltage -> Repeat until number of steps exceeded"
            n193 = local read "step interval [s]"() -> (w317:i32)
            n194 = local read "Final volts [V]"() -> (w318:dbl)
            n195 = local read "step [V]"() -> (w319:dbl)
            n196 = stacked-sequence {
              tunnel: [w339 _] -> w324
              tunnel: w319 -> [w336 w401]
              tunnel: [_ w400] -> w315
              tunnel: w318 -> [_ w399]
              tunnel: w317 -> [w327 w398]
              tunnel: [_ w397] -> w316
              tunnel: w323 -> [w338 _]
              tunnel: w322 -> [w337 _]
              tunnel: [w335 _] -> w321
              tunnel: [_ w395] -> w313
              frame #0 {
                # "Message \"Waiting for XX seconds...\""
                # "Allow to change Current (Y) axis units (Ohm, kOhm or MOhm) and representation (Linear or Logarithmic). Generate waiting message between measurements."
                n197 = Format Into String(format string="%d", w327) -> (resulting string=w332:string)  [unwired: 2 in, 1 out]
                n198 = Concatenate Strings("Waiting for  ", w332, " seconds...") -> (w328:string)
                n199 = Get Date/Time In Seconds() -> (seconds since 1Jan1904=w329:timestamp)
                n200 = To Double Precision Float(number=w329) -> (double precision float=w330:dbl)
                n201 = while {
                  tunnel: w336 -> [w348]
                  shift-left: w337 -> [w352]
                  shift-right: [w345] -> w335
                  shift-left: w338 -> [w353]
                  shift-right: [w354] -> w339
                  tunnel: w328 -> [w346]
                  tunnel: w327 -> [w358]
                  tunnel: w330 -> [w359]
                  stop <- w360 continue-if-true
                  # "\"Current status:\" indicator shows message:\n         Waiting for XX seconds...\n         Timer status: YY\"\nwhere XX is the \"step interval [s]\" and YY is\nthe time since the last measurement."
                  # "Repeats the loop if time between steps is less than \"step interval [s]\""
                  # "Loop repeated every 100 ms"
                  n202 = local read "Scales"() -> (w354:T1)
                  n203 = local read "Iscale"() -> (w345:enum16{"Ohms", "kiloOhms", "MegaOhms"})
                  n204 = Absolute Value(x=w348) -> (abs(x)=w347:dbl)
                  n205 = Get Date/Time In Seconds() -> (seconds since 1Jan1904=w344:timestamp)
                  n206 = Not Equal?(x=w352, y=w345) -> (x != y?=w343:bool)
                  n207 = Not Equal?(x=w353, y=w354) -> (x != y?=w355:bool)
                  n208 = To Double Precision Float(number=w344) -> (double precision float=w364:dbl)
                  n209 = case shown="True" w355 {
                    tunnel: w354 -> [_ w388]
                    frame False {
                    }
                    frame True {
                      # "Linear (0) or Logarithmical (1) representation of X and Y axis in IV graph"
                      n210 = case shown="..\"Lin - Lin\"" w388 {
                        tunnel: [w389 1 0 w394] -> w387
                        tunnel: [w389 0 1 w394] -> w386
                        frame .."Lin - Lin" {
                          w389 = 0
                        }
                        frame "Log - Lin" {
                        }
                        frame "Lin - Log" {
                        }
                        frame "Log - log".. {
                          w394 = 1
                        }
                      }
                      n211 = property on="Igraph" class="XYGraph (strict)"("X Scale.Mapping Mode"=w387) -> ()  [unwired: 2 in, 2 out]
                      n212 = property on="Igraph" class="XYGraph (strict)"("Y Scale.Mapping Mode"=w386, "YScale.Minimum"=w386) -> ()  [unwired: 2 in, 2 out]
                    }
                  }
                  n213 = case shown="True" w343 {
                    tunnel: w347 -> [_ _]
                    tunnel: w345 -> [_ w373]
                    frame False {
                    }
                    frame True {
                      w367 = T3."Read Array" ("Action")
                      # "Sets minimum in Current (Y) axis in 0 if linear and 1 if logarithmic"
                      # "Converts the current measurements to the units (Ohm, kOhm or MOhm) selected and updates the IV graph"
                      n214 = local read "Current reading No."() -> (w375:u32)
                      n215 = call "IVData.vi"("Action"=w367, "Array No."=u32 1 ("Action")) -> ("Array OUT"=w376:dbl[])  [unwired: 3 in, 1 out]
                      n216 = Array Subset(array=w376, index=0, length=w375) -> (w372:dbl[])
                      n217 = Absolute Value(x=w372) -> (abs(x)=w371:dbl[])
                      n218 = case shown="\"MegaOhms\".." w373 {
                        tunnel: [w379 w380 w384] -> w378
                        tunnel: w371 -> [w379 w382 w385]
                        frame .."Ohms" {
                        }
                        frame "kiloOhms" {
                          # "Converts nA to µA"
                          n219 = Divide(x=w382, y=1000.0) -> (x/y=w380:dbl[])
                        }
                        frame "MegaOhms".. {
                          # "Converts nA to mA"
                          n220 = Divide(x=w385, y=1000000.0) -> (x/y=w384:dbl[])
                        }
                      }
                      n221 = call "IVData.vi"("Action"=w367, "Array No."=u32 0 ("Action")) -> ("Array OUT"=w366:dbl[])  [unwired: 3 in, 1 out]
                      n222 = Absolute Value(x=w366) -> (abs(x)=w365:dbl[])
                      n223 = Bundle(w365, w378) -> (w374:cluster{dbl[], dbl[]})  [unwired: 1 in]
                      n224 = property on="Igraph" class="XYGraph (strict)"() -> ("YScale.Mapping Mode"=w369:u8)  [unwired: 2 in, 2 out]
                      n225 = local write "Igraph"(w374) -> ()
                      n226 = property on="Igraph" class="XYGraph (strict)"("YScale.Minimum"=w369) -> ()  [unwired: 2 in, 2 out]
                    }
                  }
                  n227 = Subtract(x=w364, y=w359) -> (x-y=w341:dbl)
                  n228 = Subtract(x=w358, y=w341) -> (x-y=w340:dbl)
                  n229 = Greater Than 0?(x=w340) -> (x > 0?=w342:bool)
                  n230 = Format Into String(format string="%d", w340) -> (resulting string=w362:string)  [unwired: 2 in, 1 out]
                  n231 = local read "abort"() -> (w357:bool)
                  n232 = Not(x=w357) -> (.not. x?=w363:bool)
                  n233 = And(x=w342, y=w363) -> (x .and. y?=w360:bool)
                  n234 = Concatenate Strings(w346, "\r\n", "Timer status: ", w362) -> (w356:string)
                  n235 = local write "STATUS 1"(w356) -> ()
                  n236 = Wait (ms)(milliseconds to wait=u32 100) -> ()  [unwired: 1 out]
                }
              }
              frame #1 {
                # "Read and Update PTP plot and T/RH with the new measurement and increment voltage for the new measurement step"
                n237 = local read "abort"() -> (w396:bool)
                n238 = case shown="False" w396 {
                  tunnel: [w407 w554] -> w397
                  tunnel: w398 -> [w406 _]
                  tunnel: w399 -> [w405 _]
                  tunnel: [w403 w554] -> w400
                  tunnel: w401 -> [w404 _]
                  tunnel: [w402 w554] -> w395
                  frame False {
                    # "\"ABORT\" button NOT pressed"
                    n239 = stacked-sequence {
                      seq-local: [w421 _ _] -> [_ w464 _]
                      seq-local: [w419 _ _] -> [_ _ w523]
                      seq-local: [w417 _ _] -> [_ _ w524]
                      tunnel: w404 -> [_ _ w529]
                      tunnel: w405 -> [_ _ w521]
                      tunnel: [_ _ w527] -> w407
                      tunnel: [_ _ w526] -> w403
                      tunnel: w406 -> [_ _ _]
                      tunnel: [w440 _ _] -> w402
                      frame #0 {
                        # "Measure current and compute \nresistance."
                        # "Write Relative Humidity [%] in 4th column"
                        # "Write Temperature [ºC] in 3rd column"
                        # "Write Resistance [Ohms] in 2nd column"
                        # "Write Voltage [V] in 1st column"
                        # "Increase in 1 the measurement number"
                        # "Convert to nA"
                        # "Show \"Reading current ...\" message \nin \"Current status:\" indicator"
                        # "Show date/time of last measurement \nin \"Last reading at:\" indicator"
                        # "READ and WRITE Voltage/Current/Temperature/Relative Humidity. Check compliance. Show date/time of last measurement and \"Reading current...\" message."
                        n240 = global read "QC_MeasurementSetup.vi" "PTP Measurement Parameters"() -> (w434:T6)
                        n241 = Get Date/Time String(want seconds? (F)=TRUE) -> (time string=w437:string)  [unwired: 2 in, 1 out]
                        n242 = local write "Last reading at:"(w437) -> ()
                        n243 = local write "STATUS 1"("Reading current ..." ("status")) -> ()
                        n244 = Unbundle By Name(w434) -> ("SMU"=w432:refnum<class "SupplyControl.lvclass">, "Set Current Limit?"=w433:bool, "Arduino"=w430:refnum<class "ArduinoControl.lvclass">, "Temperature Readout"=w431:enum16{"Read Arduino", "Enter manually"})
                        n245 = local read "Current Volts:"() -> (w416:dbl)
                        n246 = call-dynamic "Supply_ReadCurrent.vi"("SupplyControl in"=w432) -> ("error out"=w418:errorcluster, "Current in nA"=w409:dbl, "SupplyControl out"=w419:refnum<class "SupplyControl.lvclass">)  [unwired: 8 in]
                        n247 = case shown="True" w433 {
                          tunnel: [FALSE w460] -> w440
                          tunnel: w419 -> [_ w459]
                          tunnel: w418 -> [w455 w458]
                          tunnel: [w455 w457] -> w417
                          frame False {
                            # "Measurement without compliance"
                          }
                          frame True {
                            # "Current > Compliance?"
                            n248 = call-dynamic "Supply_ComplianceCheck.vi"("error in (no error)"=w458, "SupplyControl in"=w459) -> ("error out"=w457:errorcluster, "Compliance exceeded?"=w460:bool)  [unwired: 6 in, 2 out]
                          }
                        }
                        n249 = case shown="\"Read Arduino\"" w431 {
                          tunnel: [w448 w454] -> w438
                          tunnel: [w445 w453] -> w435
                          tunnel: w430 -> [_ w452]
                          frame "Enter manually", Default {
                            # "Read T/RH entered manually"
                            n250 = local read "Temp."() -> (w450:dbl[])
                            n251 = local read "RH"() -> (w446:dbl[])
                            n252 = Index Array(array=w450, index=0) -> (element=w448:dbl)
                            n253 = Index Array(array=w446, index=0) -> (element=w445:dbl)
                          }
                          frame "Read Arduino" {
                            # "Read  T/RH from Arduino"
                            n254 = call "ArduinoRead.vi"("Arduino function"=enum16{"T/RH", "Interlock", "Edgesense"}."T/RH", "ArduinoControl in"=w452) -> ("rel. Humidity [%]"=w453:dbl, "Temperature [°C]"=w454:dbl)  [unwired: 4 in, 4 out]
                          }
                        }
                        n255 = Divide(x=w409, y=10000000000.0) -> (x/y=w413:dbl)
                        n256 = Divide(x=w416, y=w413) -> (x/y=w415:dbl)
                        n257 = Absolute Value(x=w415) -> (abs(x)=w408:dbl)
                        n258 = local read "Current reading No."() -> (w410:u32)
                        n259 = local read "Current reading No."() -> (w426:u32)
                        n260 = local read "Current reading No."() -> (w420:u32)
                        n261 = local read "Current reading No."() -> (w427:u32)
                        n262 = local read "Current reading No."() -> (w428:u32)
                        n263 = call "IVData.vi"("Action"=T3."Write Element", "Array No."=u32 5, "Array Size / Index"=w410, "Data IN"=w409) -> ()  [unwired: 1 in, 2 out]
                        n264 = local read "Current reading No."() -> (w422:u32)
                        n265 = call "IVData.vi"("Action"=T3."Write Element", "Array No."=u32 2, "Array Size / Index"=w426, "Data IN"=w438) -> ()  [unwired: 1 in, 2 out]
                        n266 = call "IVData.vi"("Action"=T3."Write Element", "Array No."=u32 3, "Array Size / Index"=w420, "Data IN"=w435) -> ()  [unwired: 1 in, 2 out]
                        n267 = call "IVData.vi"("Action"=T3."Write Element", "Array No."=0, "Array Size / Index"=w428, "Data IN"=w416) -> ()  [unwired: 1 in, 2 out]
                        n268 = call "IVData.vi"("Action"=T3."Write Element", "Array No."=u32 1, "Array Size / Index"=w427, "Data IN"=w408) -> ()  [unwired: 1 in, 2 out]
                        n269 = Increment(x=w422) -> (x+1=w421:u32)
                        n270 = local write "Current reading No."(w421) -> ()
                      }
                      frame #1 {
                        w463 = T3."Read Array" ("Action")
                        w474 = u32 5 ("y")
                        # "Update Current/Voltage plots"
                        # "Set minimum in Current (Y) axis in 0 if linear and 1 if logarithmic"
                        # "Update PTP plot and show Temperature/Relative Humidity and last 5 readings of Current/Voltage"
                        n271 = call "IVData.vi"("Action"=w463) -> ("Array OUT"=w462:dbl[])  [unwired: 4 in, 1 out]
                        n272 = call "IVData.vi"("Action"=w463, "Array No."=1) -> ("Array OUT"=w476:dbl[])  [unwired: 3 in, 1 out]
                        n273 = Absolute Value(x=w462) -> (abs(x)=w461:dbl[])
                        n274 = Array Subset(array=w476, index=0, length=w464) -> (w469:dbl[])
                        n275 = Greater?(x=w464, y=w474) -> (0:w473:bool)
                        n276 = local read "Iscale"() -> (w475:enum16{"Ohms", "kiloOhms", "MegaOhms"})
                        n277 = Absolute Value(x=w469) -> (abs(x)=w468:dbl[])
                        n278 = case shown="False" w473 {
                          tunnel: w464 -> [w480 w483]
                          tunnel: w474 -> [_ w482]
                          tunnel: [w480 w482] -> w472
                          tunnel: [0 w481] -> w470
                          frame False {
                          }
                          frame True {
                            n279 = Subtract(x=w483, y=w482) -> (x-y=w481:u32)
                          }
                        }
                        n280 = property on="Igraph" class="XYGraph (strict)"() -> ("YScale.Mapping Mode"=w465:u8)  [unwired: 2 in, 2 out]
                        n281 = case shown="..\"Ohms\"" w475 {
                          tunnel: [w508 w509 w512] -> w478
                          tunnel: w468 -> [w508 w511 w514]
                          frame .."Ohms" {
                          }
                          frame "kiloOhms" {
                            # "Converts nA to µA"
                            n282 = Divide(x=w511, y=1000.0) -> (x/y=w509:dbl[])
                          }
                          frame "MegaOhms".. {
                            # "Converts nA to mA"
                            n283 = Divide(x=w514, y=1000000.0) -> (x/y=w512:dbl[])
                          }
                        }
                        n284 = property on="Igraph" class="XYGraph (strict)"("YScale.Minimum"=w465) -> ()  [unwired: 2 in, 2 out]
                        n285 = for {
                          N: 4 -> [_]
                          tunnel: w472 -> [w488]
                          tunnel: w470 -> [w487]
                          tunnel: w464 -> [w484]
                          i -> [w489]
                          # "Update \"Last 5 readings:\" PTP indicator and T/RH indicators"
                          n286 = call "IVData.vi"("Action"=T3."Read Array", "Array No."=w489) -> ("Array OUT"=w486:dbl[])  [unwired: 3 in, 1 out]
                          n287 = case shown="1" w489 {
                            tunnel: w488 -> [w492 w496 _ _]
                            tunnel: w487 -> [w493 w497 _ _]
                            tunnel: w486 -> [w491 w495 w501 w506]
                            tunnel: w484 -> [_ _ w499 w504]
                            frame ..0 {
                              # "Read Voltage from 1st column"
                              n288 = Array Subset(array=w491, index=w493, length=w492) -> (w490:dbl[])
                              n289 = local write "Volts"(w490) -> ()
                            }
                            frame 1 {
                              # "Read Current from 2nd column"
                              n290 = Array Subset(array=w495, index=w497, length=w496) -> (w494:dbl[])
                              n291 = local write "R_eff"(w494) -> ()
                            }
                            frame 2 {
                              # "Read Temperature from 3rd column"
                              n292 = Decrement(x=w499) -> (x-1=w498:u32)
                              n293 = Array Subset(array=w501, index=w498, length=1) -> (w500:dbl[])
                              n294 = local write "Temp."(w500) -> ()
                            }
                            frame 3.. {
                              # "Read Relative Humidity from 4th column"
                              n295 = Decrement(x=w504) -> (x-1=w503:u32)
                              n296 = Array Subset(array=w506, index=w503, length=1) -> (w505:dbl[])
                              n297 = local write "RH"(w505) -> ()
                            }
                          }
                        }
                        n298 = Bundle(w461, w478) -> (w466:cluster{dbl[], dbl[]})  [unwired: 1 in]
                        n299 = local write "Igraph"(w466) -> ()
                      }
                      frame #2 {
                        # "Increase volts and check for end of ramp"
                        # "Increase voltage and check compliance"
                        n300 = local read "Current Volts:"() -> (w516:dbl)
                        n301 = local read "Current Volts:"() -> (w515:dbl)
                        n302 = local read "positive ramp?"() -> (w525:bool)
                        n303 = Quotient & Remainder(x=w515, y=w521) -> (x-y*floor(x/y)=w522:dbl, floor(x/y)=w520:dbl)
                        n304 = case shown="False" w525 {
                          tunnel: w521 -> [w532 w536]
                          tunnel: w529 -> [w533 w539]
                          tunnel: [w531 w538] -> w517
                          tunnel: [w530 w535] -> w528
                          tunnel: w516 -> [w534 w537]
                          frame False {
                            n305 = Subtract(x=w534, y=w533) -> (x-y=w530:dbl)
                            n306 = Greater Or Equal?(x=w530, y=w532) -> (x >= y?=w531:bool)
                          }
                          frame True {
                            n307 = Add(x=w537, y=w539) -> (x+y=w535:dbl)
                            n308 = Less Or Equal?(x=w535, y=w536) -> (x <= y?=w538:bool)
                          }
                        }
                        n309 = Not Equal To 0?(x=w522) -> (x != 0?=w518:bool)
                        n310 = Equal To 0?(x=w520) -> (x = 0?=w519:bool)
                        n311 = Or(x=w518, y=w519) -> ()  [unwired: 1 out]
                        n312 = case shown="False" w517 {
                          tunnel: w528 -> [_ w551]
                          tunnel: [TRUE FALSE] -> w527
                          tunnel: [FALSE w542] -> w526
                          tunnel: w515 -> [_ w549]
                          tunnel: w524 -> [_ w548]
                          tunnel: w523 -> [_ w547]
                          frame False {
                          }
                          frame True {
                            # "Message \"Incrementing volts.\""
                            # "Increase  voltage, check compliance and check IV supply errors"
                            n313 = local read "step [V]"() -> (w545:dbl)
                            n314 = call "SupplyRamp.vi"("error in"=w548, "Requested Voltage"=w551, "Step Size"=w545, "Step Delay"=100, "Supply IN"=w547, "Starting Voltage"=w549) -> ("error out"=w543:errorcluster, "Compliance exceeded"=w542:bool, "Current Voltage"=w546:dbl)  [unwired: 2 in, 1 out]
                            n315 = local write "STATUS 1"("Incrementing volts.") -> ()
                            n316 = case shown="No Error" w543 {
                              tunnel: w546 -> [w553 _]
                              frame No Error {
                                n317 = local write "Current Volts:"(w553) -> ()
                              }
                              frame Error {
                              }
                            }
                            n318 = property on="Bias On/Off:" class="Bool (strict)"("Blinking"=w542) -> ()  [unwired: 2 in, 2 out]
                          }
                        }
                      }
                    }
                  }
                  frame True {
                    w554 = FALSE
                    # "\"ABORT\" button pressed"
                  }
                }
              }
            }
            n319 = case shown="False" w315 {
              frame False {
              }
              frame True {
                n320 = property on="Bias On/Off:" class="Bool (strict)"("Blinking"=TRUE) -> ()  [unwired: 2 in, 2 out]
              }
            }
            n321 = Build Array(w316, w315, "abort", w313) -> (w320:bool[])
            n322 = Or Array Elements(Boolean array=w320) -> (logical OR=w326:bool)
            n323 = Not(x=w326) -> (.not. x?=w325:bool)
          }
        }
        frame True {
          w556 = FALSE
          # "Flag compliance as reason for end of run"
          # "Compliance exceeded when first voltage applied"
          n324 = local write "STATUS 1"("Run aborted - compliance exceeded.") -> ()
          n325 = Build Array(w556, TRUE, w556, w556) -> (w557:bool[])
        }
      }
      n326 = Search 1D Array(1D array=w303, element=TRUE) -> (index of element=w301:i32)  [unwired: 1 in]
      n327 = Increment(x=w301) -> (x+1=w300:i32)
      n328 = case shown="1" w300 {
        tunnel: ["" "Run ended normally" "Compliance exceeded" "Run aborted - by user" "Run aborted - Ilimit exceeded"] -> w295
        frame ..0 {
        }
        frame 1 {
        }
        frame 2 {
        }
        frame 3 {
        }
        frame 4.. {
        }
      }
      n329 = Concatenate Strings(w295, "\r\n", "RAMPING DOWN VOLTS") -> (w298:string)
      n330 = global read "QC_RunInformation.vi" "Run info"() -> (w299:T7)
      n331 = Bundle By Name(cluster=w299, "End of Run comment:"=w295) -> (w294:T7)
      n332 = local write "STATUS 1"(w298) -> ()
      n333 = global write "QC_RunInformation.vi" "Run info"(w294) -> ()
    }
    frame #4 {
      # "Ramp down, switch off supply, ask to save data."
      n334 = stacked-sequence {
        frame #0 {
          w562 = 0.0
          # "Switch Bias supply to STANDBY"
          # "s -> ms"
          # "Switch SMU supply to STANDBY"
          # "s -> ms"
          # "Ramp down voltage and switch suppys to standby"
          n335 = global read "QC_MeasurementSetup.vi" "PTP Measurement Parameters"() -> (w578:T6)
          n336 = Unbundle By Name(w578) -> ("Bias Voltage [V]"=w563:dbl, "SMU"=w577:refnum<class "SupplyControl.lvclass">, "Ramp down Interval [s]"=w566:i32, "Test Step Size [V]"=w572:dbl, "Switching"=w573:refnum<class "Switching.lvclass">, "Matrix used?"=w574:bool, "Supply"=w567:refnum<class "SupplyControl.lvclass">, "Ramp down steps [V]"=w560:dbl)
          n337 = local read "Current Volts:"() -> (w565:dbl)
          n338 = Multiply(x=w566, y=1000) -> (x*y=w580:i32)
          n339 = call "SupplyRamp.vi"("Requested Voltage"=w562, "Step Size"=w572, "Step Delay"=w580, "Supply IN"=w577, "Starting Voltage"=w565) -> ("error out"=w576:errorcluster, "Supply OUT"=w575:refnum<class "SupplyControl.lvclass">, "Current Voltage"=w564:dbl)  [unwired: 3 in, 1 out]
          n340 = local write "Current Volts:"(w564) -> ()
          n341 = call-dynamic "Supply_Stby.vi"("error in (no error)"=w576, "SupplyControl in"=w575) -> ()  [unwired: 8 in, 2 out]
          n342 = Multiply(x=w566, y=1000) -> (x*y=w571:i32)
          n343 = call "SupplyRamp.vi"("Requested Voltage"=w562, "Step Size"=w560, "Step Delay"=w571, "Supply IN"=w567, "Starting Voltage"=w563) -> ("error out"=w569:errorcluster, "Supply OUT"=w568:refnum<class "SupplyControl.lvclass">)  [unwired: 3 in, 2 out]
          n344 = call-dynamic "Supply_Stby.vi"("error in (no error)"=w569, "SupplyControl in"=w568) -> ("error out"=w561:errorcluster)  [unwired: 8 in, 1 out]
          n345 = case shown="True" w574 {
            tunnel: w573 -> [_ w585]
            tunnel: w561 -> [_ w581]
            frame False {
            }
            frame True {
              # "CLOSE Switching Matrix"
              # "RESET Switching  Matrix"
              n346 = call-dynamic "MatrixSwitch.vi"("error in (no error)"=w581, "Action"=T4."Reset", "Switching in"=w585) -> ("error out"=w582:errorcluster, "Switching out"=w583:refnum<class "Switching.lvclass">)  [unwired: 6 in, 1 out]
              n347 = call-dynamic "Close.vi"("error in (no error)"=w582, "Switching in"=w583) -> ()  [unwired: 8 in, 2 out]
            }
          }
        }
        frame #1 {
          w590 = 0
          # "\"Current Volts\" indicator back to 0.00 V"
          # "\"Bias  On/Off\" indicator in Off (red)"
          # "\"ABORT\" button disanabled \nand dimmed (Disabled=2)"
          # "\"QUIT\" and \"Save & QUIT\" buttons \nenabled (Disabled=0)"
          # "Reset \"Current Volts\" and \"Bias On/Off\" indicators, \"ABORT\" button disabled and \"QUIT\"/\"Save & QUIT\" buttons enabled"
          n348 = property on="Quit & Save" class="Bool"("DisabledEnum"=w590) -> ()  [unwired: 2 in, 2 out]
          n349 = property on="quit (no save)" class="Bool"("DisabledEnum"=w590) -> ()  [unwired: 2 in, 2 out]
          n350 = local write "Current Volts:"(0.0 ("Current Volts:")) -> ()
          n351 = property on="abort" class="Bool (strict)"("DisabledEnum"=2) -> ()  [unwired: 2 in, 2 out]
          n352 = local write "Bias On/Off:"(FALSE ("Visible")) -> ()
          n353 = local write "STATUS 1"("Run finished. \nSave data?" ("STATUS 1")) -> ()
        }
      }
    }
    frame #5 {
      # "*WARNING*: \"Done!\" indicator in \nFront Panel hidden."
      # "Switch off Arduino if used for T/RH measurement"
      # "Display and save data"
      n354 = global read "QC_MeasurementSetup.vi" "PTP Measurement Parameters"() -> (w599:T6)
      n355 = local read "Scales"() -> (w601:T1)
      n356 = local read "Iscale"() -> (w600:enum16{"Ohms", "kiloOhms", "MegaOhms"})
      n357 = while {
        shift-left: w600 -> [w632]
        shift-right: [w631] -> _
        shift-left: w601 -> [w634]
        shift-right: [w633] -> _
        tunnel: ["Quit & Save"] -> w603
        tunnel: ["quit (no save)"] -> w602
        stop <- w629 continue-if-true
        # "Loop and await decision on whether to save or junk data"
        n358 = local read "Scales"() -> (w633:T1)
        n359 = local read "Iscale"() -> (w631:enum16{"Ohms", "kiloOhms", "MegaOhms"})
        n360 = Not Equal?(x=w634, y=w633) -> (x != y?=w627:bool)
        n361 = Not Equal?(x=w632, y=w631) -> (x != y?=w626:bool)
        n362 = case shown="True" w627 {
          tunnel: w633 -> [_ w659]
          frame False {
          }
          frame True {
            # "Allow to change the IV plot representation (Linear=0, Logarithmic=1)"
            n363 = case shown="..\"Lin - Lin\"" w659 {
              tunnel: [w660 1 0 w665] -> w658
              tunnel: [w660 0 1 w665] -> w657
              frame .."Lin - Lin" {
                w660 = 0
              }
              frame "Log - Lin" {
              }
              frame "Lin - Log" {
              }
              frame "Log - log".. {
                w665 = 1
              }
            }
            n364 = property on="Igraph" class="XYGraph (strict)"("X Scale.Mapping Mode"=w658) -> ()  [unwired: 2 in, 2 out]
            n365 = property on="Igraph" class="XYGraph (strict)"("Y Scale.Mapping Mode"=w657, "YScale.Minimum"=w657) -> ()  [unwired: 2 in, 2 out]
          }
        }
        n366 = case shown="True" w626 {
          tunnel: w631 -> [_ w645]
          frame False {
          }
          frame True {
            w638 = T3."Read Array" ("Action")
            # "Set minimum in Current (Y) axis in 0 if linear and 1 if logarithmic"
            # "Allow to change the Y Scale (Ohms, kiloOhms, MegaOhms)"
            n367 = global read "QC_MeasurementSetup.vi" "PTP Measurement Parameters"() -> (w640:T6)
            n368 = property on="Igraph" class="XYGraph (strict)"() -> ("YScale.Mapping Mode"=w641:u8)  [unwired: 2 in, 2 out]
            n369 = property on="Igraph" class="XYGraph (strict)"("YScale.Minimum"=w641) -> ()  [unwired: 2 in, 2 out]
            n370 = Unbundle By Name(w640) -> ("Test Number of Steps"=w635:u32)
            n371 = call "IVData.vi"("Action"=w638, "Array No."=u32 1 ("Action")) -> ("Array OUT"=w647:dbl[])  [unwired: 3 in, 1 out]
            n372 = Array Subset(array=w647, index=0, length=w635) -> (w644:dbl[])
            n373 = Absolute Value(x=w644) -> (abs(x)=w643:dbl[])
            n374 = call "IVData.vi"("Action"=w638, "Array No."=u32 0 ("Action")) -> ("Array OUT"=w637:dbl[])  [unwired: 3 in, 1 out]
            n375 = case shown="\"kiloOhms\"" w645 {
              tunnel: [w650 w651 w655] -> w649
              tunnel: w643 -> [w650 w653 w656]
              frame .."Ohms" {
              }
              frame "kiloOhms" {
                n376 = Divide(x=w653, y=1000.0) -> (x/y=w651:dbl[])
              }
              frame "MegaOhms".. {
                n377 = Divide(x=w656, y=1000000.0) -> (x/y=w655:dbl[])
              }
            }
            n378 = Absolute Value(x=w637) -> (abs(x)=w636:dbl[])
            n379 = Bundle(w636, w649) -> (w646:cluster{dbl[], dbl[]})  [unwired: 1 in]
            n380 = local write "Igraph"(w646) -> ()
          }
        }
        n381 = Not Or(1:"quit (no save)", 2:"Quit & Save") -> (0:w629:bool)
      }
      n382 = Unbundle By Name(w599) -> ("Temperature Readout"=w598:enum16{"Read Arduino", "Enter manually"}, "Arduino"=w592:refnum<class "ArduinoControl.lvclass">)
      n383 = case shown="\"Read Arduino\"" w598 {
        tunnel: w592 -> [_ w625]
        frame "Enter manually", Default {
        }
        frame "Read Arduino" {
          n384 = call "ArduinoClose.vi"("ArduinoControl in"=w625) -> ()  [unwired: 9 in, 2 out]
        }
      }
      n385 = case shown="True" w602 {
        tunnel: [FALSE w667] -> w604
        frame False {
        }
        frame True {
          n386 = Two Button Dialog(message="Are you sure you don't want to save the data?", 1:"Quit" ("F button name (\"Cancel\")"), 2:"Save data" ("T button name (\"OK\")")) -> (T button?=w667:bool)
        }
      }
      n387 = Or(x=w603, y=w604) -> (x .or. y?=w597:bool)
      n388 = flat-sequence {
        tunnel: w597 -> [w605]
        tunnel: [w605] -> w593
        tunnel: [TRUE] -> w591
        frame #0 {
          n389 = case shown="True" w605 {
            frame False {
            }
            frame True {
              w608 = T3."Read Array" ("Action")
              # "Show \"Saving Data ...\" message"
              # "Save data in file"
              n390 = local write "STATUS 1"("Saving Data ...") -> ()
              n391 = call "IVData.vi"("Action"=w608, "Array No."=u32 0 ("Action")) -> ("Array OUT"=w617:dbl[])  [unwired: 3 in, 1 out]
              n392 = call "IVData.vi"("Action"=w608, "Array No."=u32 1 ("Action")) -> ("Array OUT"=w616:dbl[])  [unwired: 3 in, 1 out]
              n393 = call "IVData.vi"("Action"=w608, "Array No."=u32 5) -> ("Array OUT"=w610:dbl[])  [unwired: 3 in, 1 out]
              n394 = Build Array(w617, w616, w610) -> (w615:dbl[][])
              n395 = Transpose 2D Array(2D array=w615) -> (transposed array=w614:dbl[][])
              n396 = call "IVData.vi"("Action"=w608, "Array No."=u32 2 ("Action")) -> ("Array OUT"=w623:dbl[])  [unwired: 3 in, 1 out]
              n397 = call "IVData.vi"("Action"=w608, "Array No."=u32 3 ("Action")) -> ("Array OUT"=w622:dbl[])  [unwired: 3 in, 1 out]
              n398 = call <vilib>:"Std Deviation and Variance.vi"("X"=w623) -> ("mean"=w612:dbl)  [unwired: 1 in, 2 out]
              n399 = call <vilib>:"Std Deviation and Variance.vi"("X"=w622) -> ("mean"=w613:dbl)  [unwired: 1 in, 2 out]
              n400 = call "SaveDataFile.vi"("Data Array"=w614, "Temperature"=w613, "Humidity"=w612, "Array Titles"="Voltage[V] Resistance[Ohms] Current[nA]", "Strip Segment"="") -> ()  [unwired: 7 in, 4 out]
            }
          }
        }
      }
      n401 = Select(t="Run finished.\nData saved." ("STATUS 1"), s=w593, f="Run finished.\nData not saved." ("STATUS 1")) -> (s? t:f=w596:string)
      n402 = local write "STATUS 1"(w596) -> ()
      "Done!" <- w591
    }
  }
